vi "Adjust GObject Alignment - Horizontal Center - AutoCenter.vi"(4 "error in":errorcluster, 7 "GObj Refs":refnum<vi>[](array[refnum])) -> (0 "error out":errorcluster, 3 "dup GObj Refs":refnum<vi>[](array[refnum]))   [LabVIEW 2018]
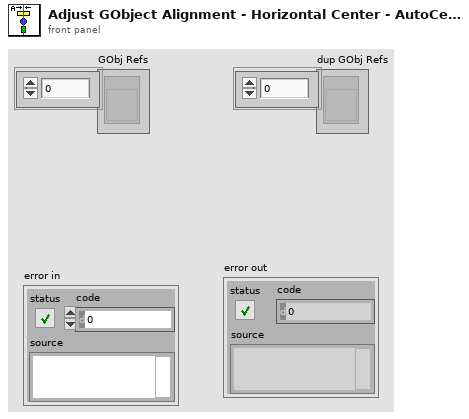
[diagram p1: front panel]
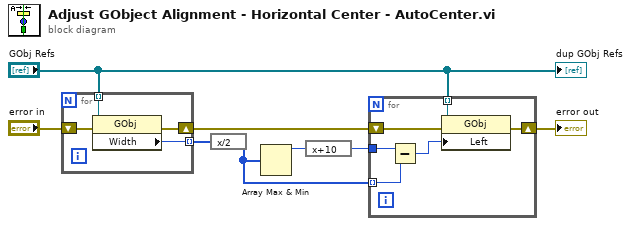
[diagram p0: block diagram]
diagram:
  n1 = for {
    tunnel: "GObj Refs" -> [w10] mode=indexing
    shift-right: [w9] -> w6
    shift-left: "error in" -> [w11]
    tunnel: [w8] -> w4 mode=indexing
    n2 = property class="GObj"(reference=w10, error in=w11) -> (error out=w9:errorcluster, "Width"=w8:u32)  [unwired: 1 out]
  }
  "error out" <- w6
  n3 = expression code="x/2"(w4) -> (w1:u32[])
  n4 = Array Max & Min(array=w1) -> (max value=w2:u32)  [unwired: 3 out]
  n5 = expression code="x+10"(w2) -> (w3:u32)
  n6 = for {
    shift-right: [w17] -> _
    shift-left: _ -> [w13]
    tunnel: w3 -> [w16]
    tunnel: "GObj Refs" -> [w14] mode=indexing
    tunnel: w1 -> [w15] mode=indexing
    n7 = Subtract(x=w16, y=w15) -> (x-y=w12:u32)
    n8 = property class="GObj"(reference=w14, error in=w13, "Left"=w12) -> (error out=w17:errorcluster)  [unwired: 1 out]
  }
  "dup GObj Refs" <- "GObj Refs"
